vi "poly_dialog_interrupt_3btn.vi"(4 "Allow user to close window? (TRUE)":bool=TRUE, 5 "Justify Message (Left)":enum16{"Left", "Center", "Right"}(ring), 6 "Keyboard Shortcuts (Left is <Enter>)":T3={"Left Button Key Shortcut"={"Control"=FALSE, "Shift"=FALSE, "Key"="<Enter>"}, "Center Button Key Shortcut"={"Control"=FALSE, "Shift"=FALSE, "Key"=""}, "Right Button Key Shortcut"={"Control"=FALSE, "Shift"=FALSE, "Key"=""}}, 7 "Window Title (\"\")":string, 8 "error in":errorcluster caption="Error in (no error)", 10 "message":string) -> (0 "error out":errorcluster, 2 "Which Button?":T2(ring)=enum."Center Button")   [LabVIEW 2015]
panel:
  in  "Button Texts (Yes, No, Cancel)":T1={"Left"="Yes", "Center"="No", "Right"="Cancel"}
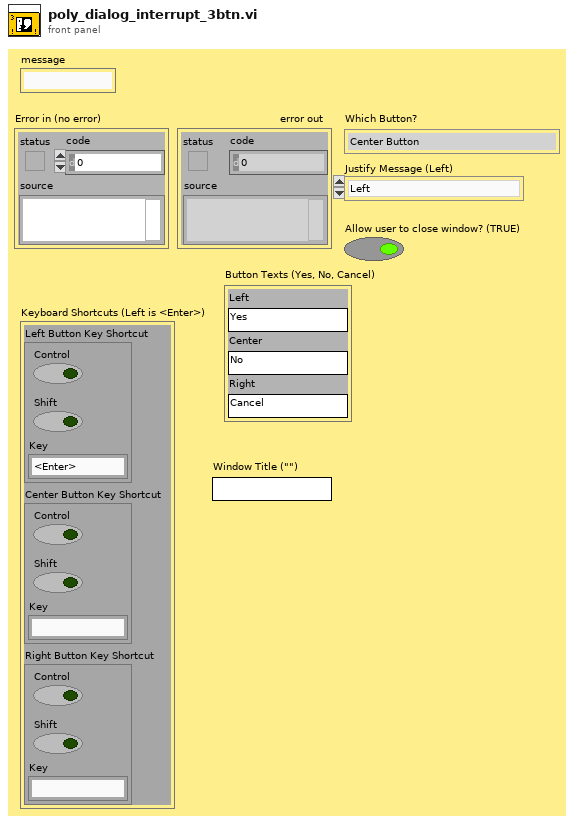
[diagram p1: front panel]
types:
  T1 = cluster{"Left":string, "Center":string, "Right":string}
  T2 = enum16{"Left Button", "Center Button", "Right Button", "Window Close"}
  T3 = cluster{"Left Button Key Shortcut":cluster{"Control":bool, "Shift":bool, "Key":string}, "Center Button Key Shortcut":cluster{"Control":bool, "Shift":bool, "Key":string}, "Right Button Key Shortcut":cluster{"Control":bool, "Shift":bool, "Key":string}}
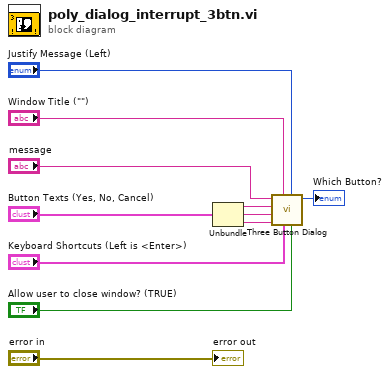
[diagram p0: block diagram]
diagram:
  n1 = Unbundle("Button Texts (Yes, No, Cancel)") -> ("Left"=w3:string, "Center"=w2:string, "Right"=w1:string)
  n2 = call <vilib>:"Three Button Dialog.vi"("Allow user to close window? (TRUE)"="Allow user to close window? (TRUE)", "Justify Message (Left)"="Justify Message (Left)", "Keyboard Shortcuts (Left is <Enter>)"="Keyboard Shortcuts (Left is <Enter>)", "Window Title (\"\")"="Window Title (\"\")", "Right Button Text (\"Cancel\")"=w1, "Center Button Text (\"No\")"=w2, "Left Button Text (\"Yes\")"=w3, "message"="message") -> ("Which Button?"=→"Which Button?":T2)  [unwired: 3 in]
  "error out" <- "error in"
